vi "PWM_FPGA (SubVI).vi"(8 "FPGA I/O In":refnum<k21>="Mod1/DO1", 11 "PWM_IN_gen":u32) -> ()   [LabVIEW 2021]
uses:
  <vilib>/eio/EIONode/EIONode.xnode
  <vilib>/rvi/eio/common/nirviEmuTemplateMethod_errors.vi
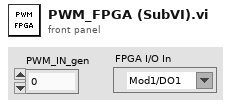
[diagram p1: front panel]
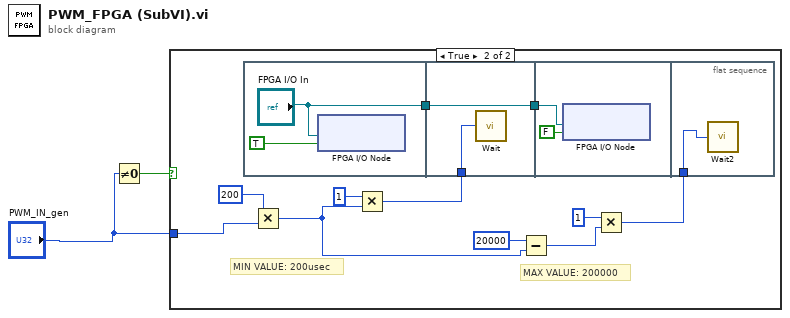
[diagram p0: block diagram]
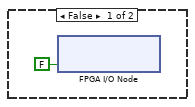
[diagram p2: hidden frame]
diagram:
  n1 = Not Equal To 0?(x="PWM_IN_gen") -> (x != 0?=w1:bool)
  n2 = case shown="True" w1 {
    tunnel: "PWM_IN_gen" -> [_ w14]
    frame False {
      n3 = xnode "FPGA I/O Node"("Mod1/DO1"=FALSE ("Mod1/DO0")) -> ()  [unwired: 1 in, 1 out]
    }
    frame True {
      # "MAX VALUE: 200000"
      # "MIN VALUE: 200usec"
      n4 = flat-sequence {
        tunnel: ["FPGA I/O In"] -> w4
        tunnel: w9 -> [w18]
        tunnel: [w17] -> w5
        tunnel: w4 -> [w17]
        tunnel: w5 -> [w19]
        tunnel: w7 -> [w21]
        frame #0 {
          n5 = xnode "FPGA I/O Node"("I/O Item"=TRUE ("Mod1/DO0"), "FPGA I/O In"="FPGA I/O In") -> ()  [unwired: 1 out]
        }
        frame #1 {
          n6 = call "Wait"("Count(uSec)"=w18) -> ()  [unwired: 1 out]
        }
        frame #2 {
          n7 = xnode "FPGA I/O Node"("I/O Item"=FALSE ("Mod1/DO0"), "FPGA I/O In"=w19) -> ()  [unwired: 1 out]
        }
        frame #3 {
          n8 = call "Wait2"("Count(uSec)"=w21) -> ()  [unwired: 1 out]
        }
      }
      n9 = Multiply(x=u32 200, y=w14) -> (x*y=w11:u32)
      n10 = Multiply(x=u32 1, y=w11) -> (x*y=w9:u32)
      n11 = Subtract(x=u32 20000, y=w11) -> (x-y=w8:u32)
      n12 = Multiply(x=u32 1, y=w8) -> (x*y=w7:u32)
    }
  }
